vi "SwerveAssistStrafe.vi"(1 "In Deadband":bool, 3 "Joystick X":dbl, 4 "Joystick Y":dbl, 9 "Strafe PID":T2={"Kp"=0.1, "Ki"=0.1, "Kd"=0.1, "N-Diff"=10, "N-Int"=20, "Int Error Window"=0.5, "Max Ouput"=1.0, "Min Output"=-1.0, "Square Derivative"=FALSE, "N-Prop"=1} {"N-Prop" min=1; "Int Error Window" min=0.0; "N-Int" min=2; "N-Diff" min=2; "Kd" min=0.0; "Ki" min=0.0; "Kp" min=0.0}, 10 "Locked X (in)":dbl format="%#_13g", 12 "Locked Y (in)":dbl format="%#_13g", 14 "Orientation Mode":enum16{"Robot-Oriented", "Field-Oriented"}(ring)) -> (20 "Strafe PID Plot":T1, 21 "In Deadband":bool, 23 "Assisted X":dbl, 24 "Assisted Y":dbl, 25 "Current Y Error (in)":dbl, 26 "Current X Error (in)":dbl, 27 "Strafe Assist On":bool)   [LabVIEW 2023]
doc: "Runs a PID controller to maintain the robot's postion relative to a vector parallel to the field's x-axis. If no goal y position is given, the driver commands are passed through unaltered."
uses:
  cf937340-f4c0-4e6b-bd78-ef74acd66303.vi
  af15fe63-c48f-490d-b061-1826781410b4.vi
  GlobalPoseAndTargeting.vi
  GlobalDriverStationCommands.vi
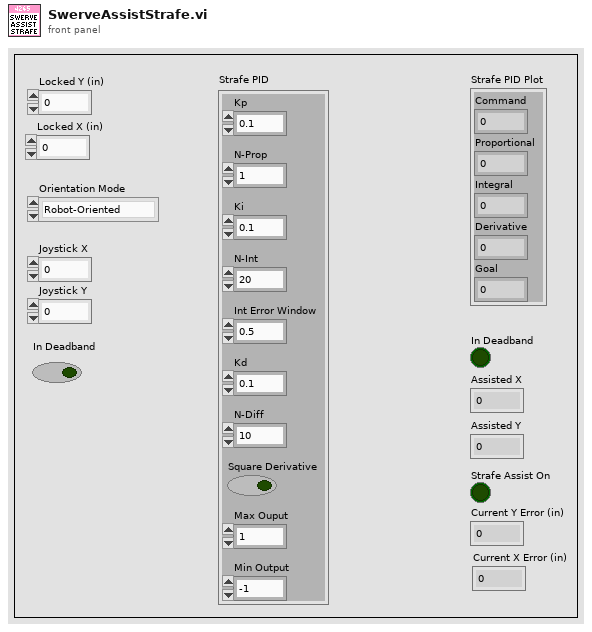
[diagram p1: front panel]
types:
  T1 = cluster{"Command":dbl, "Proportional":dbl, "Integral":dbl, "Derivative":dbl, "Goal":dbl}
  T2 = cluster{"Kp":dbl, "Ki":dbl, "Kd":dbl, "N-Diff":i32, "N-Int":i32, "Int Error Window":dbl, "Max Ouput":dbl, "Min Output":dbl, "Square Derivative":bool, "N-Prop":i32}
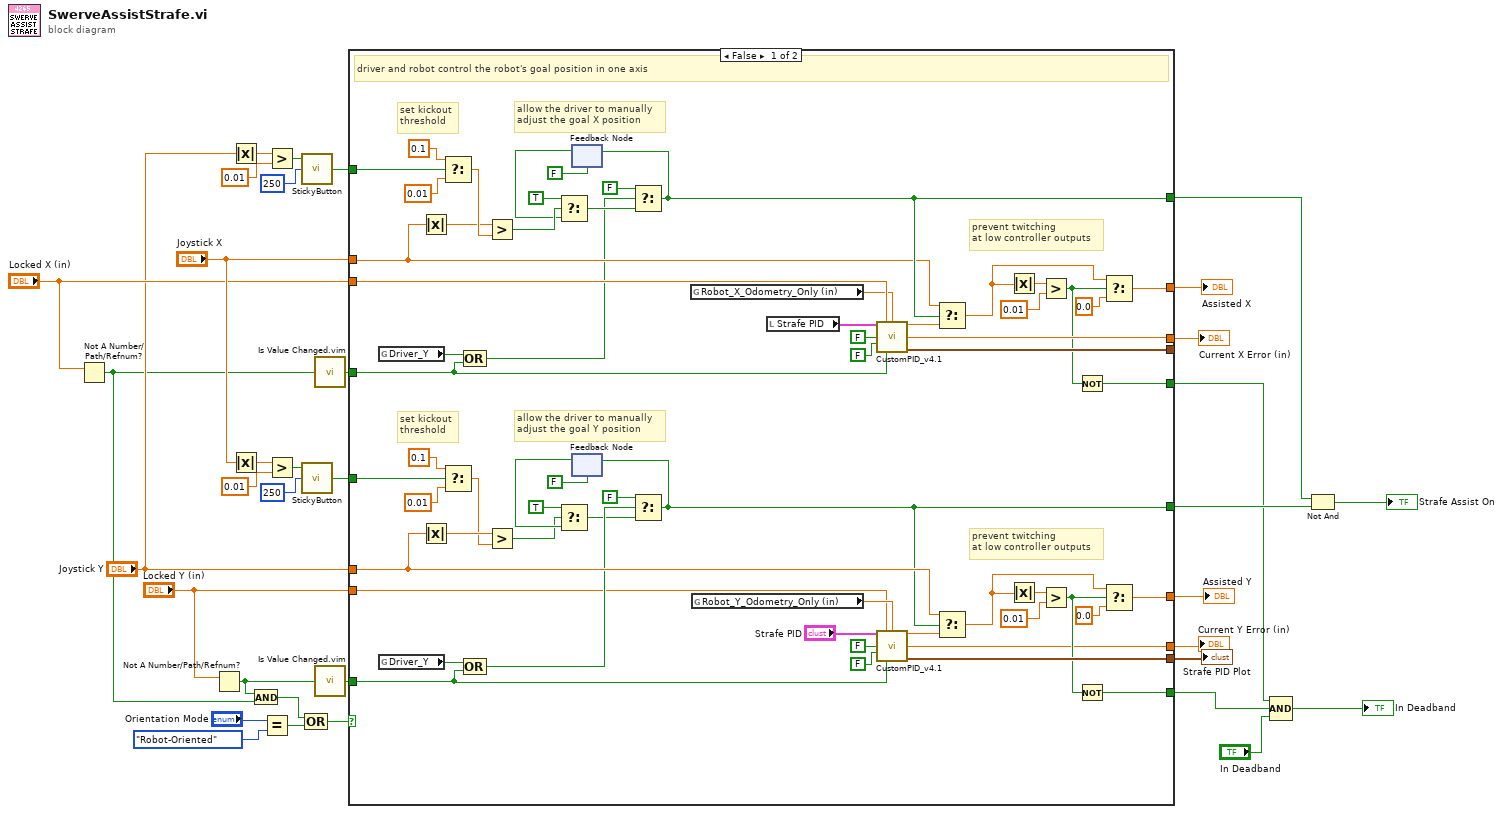
[diagram p0: block diagram]
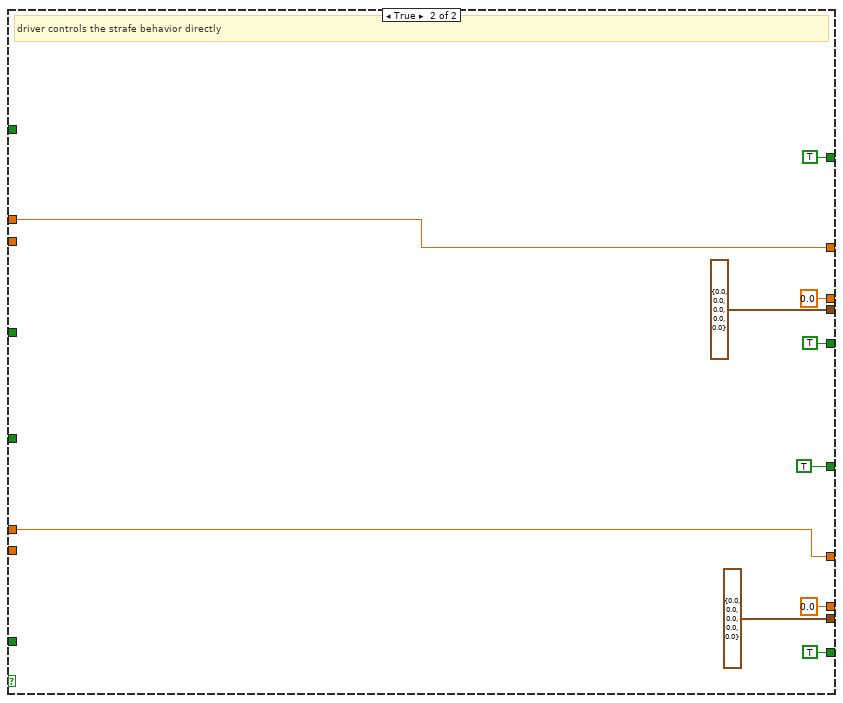
[diagram p2: hidden frame]
diagram:
  n1 = Not A Number/Path/Refnum?(number/path/refnum="Locked X (in)") -> (NaN/Path/Refnum?=w3:bool)
  n2 = Not A Number/Path/Refnum?(number/path/refnum="Locked Y (in)") -> (NaN/Path/Refnum?=w1:bool)
  n3 = Absolute Value(x="Joystick Y") -> (abs(x)=w18:dbl)
  n4 = Absolute Value(x="Joystick X") -> (abs(x)=w22:dbl)
  n5 = And(x=w1, y=w3) -> (x .and. y?=w2:bool)
  n6 = Equal?(x="Orientation Mode", y=enum16{"Robot-Oriented", "Field-Oriented"}."Robot-Oriented") -> (x = y?=w29:bool)
  n7 = Greater?(x=w18, y=0.01) -> (0:w16:bool)
  n8 = Greater?(x=w22, y=0.01) -> (0:w25:bool)
  n9 = call "StickyButton.vi"("Time threshold (ms)"=u32 250, "Button Input"=w16) -> ("Sticky Button"=w14:bool)  [unwired: 1 in]
  n10 = call "StickyButton.vi"("Time threshold (ms)"=u32 250, "Button Input"=w25) -> ("Sticky Button"=w24:bool)  [unwired: 1 in]
  n11 = Compound Arithmetic op=OR(w2, w29) -> (w4:bool)
  n12 = call "Is Value Changed.vim"("value"=w3) -> ("changed or first call?"=w19:bool)
  n13 = call "Is Value Changed.vim"("value"=w1) -> ("changed or first call?"=w35:bool)
  n14 = case shown="False" w4 {
    tunnel: "Locked Y (in)" -> [w68 _]
    tunnel: [w95 T1 {"Command"=0.0, "Proportional"=0.0, "Integral"=0.0, "Derivative"=0.0, "Goal"=0.0} ("Controller Summary")] -> w32
    tunnel: [w91 w105] -> w31
    tunnel: w35 -> [w85 _]
    tunnel: [w73 TRUE] -> w10
    tunnel: "Joystick Y" -> [w86 w105]
    tunnel: "Joystick X" -> [w65 w102]
    tunnel: [w66 0.0 ("Current Error")] -> w11
    tunnel: w24 -> [w72 _]
    tunnel: [w70 0.0 ("Current Error")] -> w21
    tunnel: "Locked X (in)" -> [w64 _]
    tunnel: w19 -> [w63 _]
    tunnel: w14 -> [w62 _]
    tunnel: [w61 T1 {"Command"=0.0, "Proportional"=0.0, "Integral"=0.0, "Derivative"=0.0, "Goal"=0.0} ("Controller Summary")] -> _
    tunnel: [w60 w102] -> w12
    tunnel: [w67 TRUE] -> w9
    tunnel: [w59 TRUE] -> w6
    tunnel: [w58 TRUE] -> w5
    frame False {
      # "set kickout\nthreshold"
      # "allow the driver to manually\nadjust the goal X position"
      # "prevent twitching\nat low controller outputs"
      # "set kickout\nthreshold"
      # "allow the driver to manually\nadjust the goal Y position"
      # "prevent twitching\nat low controller outputs"
      # "driver and robot control the robot's goal position in one axis"
      n15 = global read "GlobalDriverStationCommands.vi" "Driver_Y"() -> (w56:bool)
      n16 = global read "GlobalDriverStationCommands.vi" "Driver_Y"() -> (w71:bool)
      n17 = Absolute Value(x=w65) -> (abs(x)=w45:dbl)
      n18 = Absolute Value(x=w86) -> (abs(x)=w84:dbl)
      n19 = Select(t=0.1 ("y"), s=w62, f=0.01) -> (s? t:f=w53:dbl)
      n20 = Select(t=0.1 ("y"), s=w72, f=0.01) -> (s? t:f=w76:dbl)
      n21 = Compound Arithmetic op=OR(w56, w63) -> (w47:bool)
      n22 = Compound Arithmetic op=OR(w71, w85) -> (w82:bool)
      n23 = Greater?(x=w45, y=w53) -> (0:w50:bool)
      n24 = Greater?(x=w84, y=w76) -> (0:w79:bool)
      n25 = feedback #1(FALSE) -> (w49:bool)
      n26 = Select(t=TRUE, s=w50, f=w49) -> (s? t:f=w48:bool)
      n27 = feedback #2(FALSE) -> (w80:bool)
      n28 = Select(t=TRUE, s=w79, f=w80) -> (s? t:f=w81:bool)
      n29 = Select(t=FALSE, s=w47, f=w48) -> (s? t:f=w67:bool)
      n30 = feedback-in #1(w67) -> ()
      n31 = Select(t=FALSE, s=w82, f=w81) -> (s? t:f=w73:bool)
      n32 = feedback-in #2(w73) -> ()
      n33 = global read "GlobalPoseAndTargeting.vi" "Robot_X_Odometry_Only (in)"() -> (w57:dbl)
      n34 = global read "GlobalPoseAndTargeting.vi" "Robot_Y_Odometry_Only (in)"() -> (w69:dbl)
      n35 = local read "Strafe PID"() -> (w36:T2)
      n36 = call "CustomPID_v4.1.vi"("PID Tuning Parameters"=w36, "Goal"=w64, "Process Variable"=w57, "Reset on Goal Change ?"=FALSE, "Use Custom Error Calculation ?"=FALSE, "Reinit"=w63) -> ("Command"=w43:dbl, "Current Error"=w66:dbl, "Controller Summary"=w61:T1)  [unwired: 6 in, 1 out]
      n37 = call "CustomPID_v4.1.vi"("PID Tuning Parameters"="Strafe PID", "Goal"=w68, "Process Variable"=w69, "Reset on Goal Change ?"=FALSE, "Use Custom Error Calculation ?"=FALSE, "Reinit"=w85) -> ("Command"=w88:dbl, "Current Error"=w70:dbl, "Controller Summary"=w95:T1)  [unwired: 6 in, 1 out]
      n38 = Select(t=w65, s=w67, f=w43) -> (s? t:f=w44:dbl)
      n39 = Select(t=w86, s=w73, f=w88) -> (s? t:f=w87:dbl)
      n40 = Absolute Value(x=w44) -> (abs(x)=w39:dbl)
      n41 = Absolute Value(x=w87) -> (abs(x)=w94:dbl)
      n42 = Greater?(x=w39, y=0.01) -> (0:w42:bool)
      n43 = Greater?(x=w94, y=0.01) -> (0:w89:bool)
      n44 = Not(x=w42) -> (.not. x?=w58:bool)
      n45 = Not(x=w89) -> (.not. x?=w59:bool)
      n46 = Select(t=w44, s=w42, f=0.0 ("t")) -> (s? t:f=w60:dbl)
      n47 = Select(t=w87, s=w89, f=0.0 ("t")) -> (s? t:f=w91:dbl)
    }
    frame True {
      # "driver controls the strafe behavior directly"
    }
  }
  "Assisted X" <- w12
  "Strafe PID Plot" <- w32
  "Assisted Y" <- w31
  "Current Y Error (in)" <- w21
  "Current X Error (in)" <- w11
  n48 = Compound Arithmetic op=AND(w5, w6, "In Deadband") -> (→"In Deadband":bool)
  n49 = Not And(1:w10, 2:w9) -> (0:→"Strafe Assist On":bool)
